vi "步进电机初始化.vi"(1 "Z轴速度":dbl, 2 "Y轴速度":dbl, 3 "回零速度":dbl, 4 "细分设置":dbl, 5 "X轴速度":dbl, 6 "串口通信端口":refnum<visa-resource-name>) -> (0 "字符串":string)   [LabVIEW 2016]
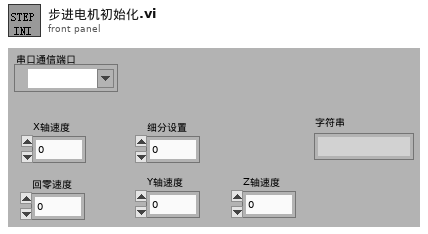
[diagram p1: front panel]
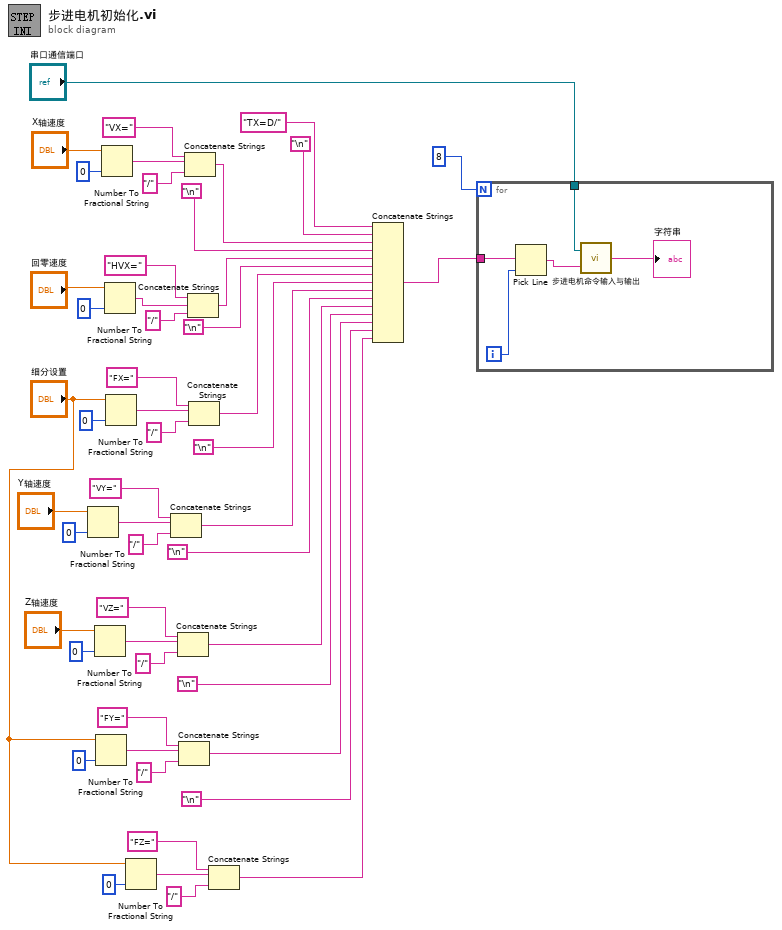
[diagram p0: block diagram]
diagram:
  n1 = Number To Fractional String(number="Y轴速度", precision (6)=i16 0 ("精度(6)")) -> (F-format string=w23:string)  [unwired: 2 out]
  n2 = Number To Fractional String(number="Z轴速度", precision (6)=i16 0 ("精度(6)")) -> (F-format string=w16:string)  [unwired: 2 out]
  n3 = Number To Fractional String(number="细分设置", precision (6)=i16 0 ("精度(6)")) -> (F-format string=w11:string)  [unwired: 2 out]
  n4 = Number To Fractional String(number="X轴速度", precision (6)=i16 0 ("精度(6)")) -> (F-format string=w48:string)  [unwired: 2 out]
  n5 = Number To Fractional String(number="回零速度", precision (6)=i16 0 ("精度(6)")) -> (F-format string=w31:string)  [unwired: 2 out]
  n6 = Number To Fractional String(number="细分设置", precision (6)=i16 0 ("精度(6)")) -> (F-format string=w40:string)  [unwired: 2 out]
  n7 = Number To Fractional String(number="细分设置", precision (6)=i16 0 ("精度(6)")) -> (F-format string=w6:string)  [unwired: 2 out]
  n8 = Concatenate Strings("VY=" ("字符串"), w23, "/" ("字符串")) -> (w21:string)
  n9 = Concatenate Strings("VZ=" ("字符串"), w16, "/" ("字符串")) -> (w14:string)
  n10 = Concatenate Strings("FY=" ("字符串"), w11, "/" ("字符串")) -> (w9:string)
  n11 = Concatenate Strings("VX=" ("字符串"), w48, "/" ("字符串")) -> (w36:string)
  n12 = Concatenate Strings("HVX=" ("字符串"), w31, "/" ("字符串")) -> (w30:string)
  n13 = Concatenate Strings("FX=" ("字符串"), w40, "/" ("字符串")) -> (w28:string)
  n14 = Concatenate Strings("FZ=" ("字符串"), w6, "/" ("字符串")) -> (w3:string)
  n15 = Concatenate Strings("TX=D/" ("字符串"), "\n", w36, "\n", w30, "\n", w28, "\n", w21, "\n", w14, "\n", w9, "\n", w3) -> (w32:string)
  n16 = for {
    N: 8 -> [_]
    tunnel: "串口通信端口" -> [w56]
    tunnel: w32 -> [w54]
    i -> [w55]
    n17 = Pick Line(multi-line string=w54, line index=w55) -> (output string=w53:string)  [unwired: 1 out]
    n18 = call "步进电机命令输入与输出.vi"("输入字符串"=w53, "串口通信端口"=w56) -> ("返回字符串"=→"字符串":string)
  }
